vi "Parse Multilines Value.vi"(8 "error in (no error)":errorcluster, 11 "String":string) -> (0 "error out":errorcluster, 2 "Value":variant, 3 "Remaining String":string)   [LabVIEW 2015, in "YAML Parser.lvclass"]
uses:
  YAML Parser.lvclass
panel:
  out "length first line":i32
  out "Lines":i32
  out "lengths":i32[](array[numeric])
  out "total length":i32
  out "First Line Value":string
  out "Key":string
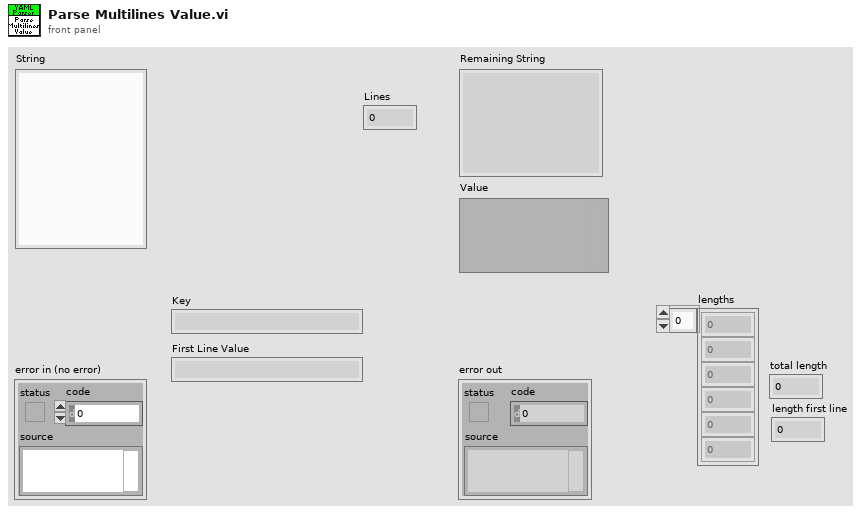
[diagram p1: front panel]
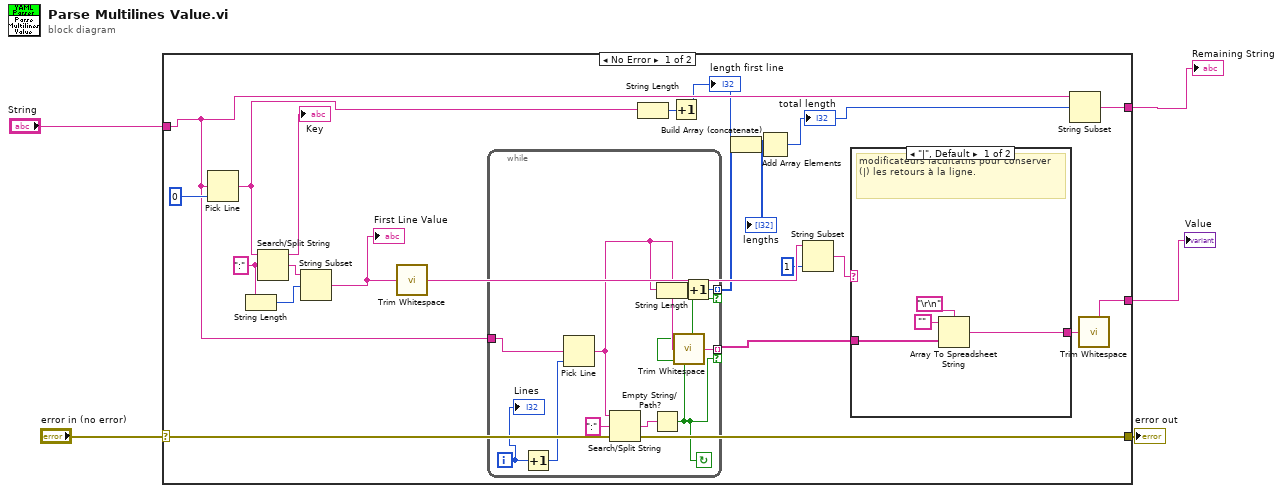
[diagram p0: block diagram]
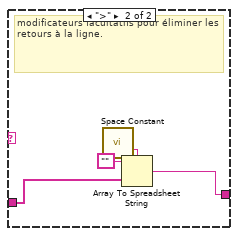
[diagram p2: hidden frame]
diagram:
  n1 = case shown="No Error" "error in (no error)" {
    selector: "error in (no error)" -> [w26 w46]
    tunnel: [w26 w46] -> w4
    tunnel: "String" -> [w13 w45]
    tunnel: [w12 w45] -> w2
    tunnel: [w6 _] -> w1
    frame No Error {
      w23 = ":" ("search string/char (-)")
      n2 = Pick Line(multi-line string=w13, line index=0) -> (output string=w16:string)  [unwired: 1 in]
      n3 = String Length(string=w23) -> (length=w22:i32)
      n4 = Search/Split String(string=w16, search string/char (-)=w23) -> (substring before match=→"Key":string, match + rest of string=w24:string)  [unwired: 1 in, 1 out]
      n5 = String Subset(string=w24, offset (0)=w22) -> (substring=w21:string)  [unwired: 1 in]
      "First Line Value" <- w21
      n6 = call <vilib>:"Trim Whitespace.vi"("string"=w21) -> ("trimmed string"=w20:string)  [unwired: 1 in]
      n7 = while {
        tunnel: w13 -> [w36]
        tunnel: [w27] -> w14 mode=indexing if=w29
        tunnel: [w33] -> w9 mode=indexing if=w29
        i -> [w28]
        stop <- w29 continue-if-true
        n8 = Increment(x=w28) -> (x+1=w35:i32)
        n9 = Pick Line(multi-line string=w36, line index=w35) -> (output string=w32:string)  [unwired: 1 in]
        n10 = Search/Split String(string=w32, search string/char (-)=":") -> (match + rest of string=w30:string)  [unwired: 1 in, 2 out]
        n11 = Empty String/Path?(string/path=w30) -> (empty?=w29:bool)
        n12 = String Length(string=w32) -> (length=w34:i32)
        n13 = call <vilib>:"Trim Whitespace.vi"("string"=w32) -> ("trimmed string"=w33:string)  [unwired: 1 in]
        n14 = Increment(x=w34) -> (x+1=w27:i32)
        "Lines" <- w28
      }
      n15 = String Length(string=w16) -> (length=w15:i32)
      n16 = Increment(x=w15) -> (x+1=w7:i32)
      "length first line" <- w7
      n17 = Build Array (concatenate)(w7, w14) -> (w11:i32[])
      "lengths" <- w11
      n18 = Add Array Elements(numeric array=w11) -> (sum=w10:i32)
      "total length" <- w10
      n19 = String Subset(string=w20, length (rest)=1 ("length (rest)")) -> (substring=w18:string)  [unwired: 1 in]
      n20 = case shown="\"|\", Default" w18 {
        tunnel: w9 -> [w38 w42]
        tunnel: [w37 w41] -> w8
        frame "|", Default {
          # "modificateurs facultatifs pour conserver (|) les retours à la ligne."
          n21 = Array To Spreadsheet String(delimiter (Tab)="\r\n", array=w38, 3:"") -> (spreadsheet string=w37:string)
        }
        frame ">" {
          # "modificateurs facultatifs pour éliminer les retours à la ligne."
          n22 = call <vilib>:"Space Constant.vi"() -> ("String"=w43:string)
          n23 = Array To Spreadsheet String(delimiter (Tab)=w43, array=w42, 3:"") -> (spreadsheet string=w41:string)
        }
      }
      n24 = String Subset(string=w13, offset (0)=w10) -> (substring=w12:string)  [unwired: 1 in]
      n25 = call <vilib>:"Trim Whitespace.vi"("string"=w8) -> ("trimmed string"=w6:string)  [unwired: 1 in]
    }
    frame Error {
    }
  }
  "error out" <- w4
  "Value" <- w1
  "Remaining String" <- w2
